vi "VelocityModeTestSDI.vi"() -> ()   [LabVIEW 2014]
uses:
  <resource>/objmgr/nimcca.rc
panel:
  in  "Velocity Setpoint":dbl
  in  "stop":bool
  out "error out":errorcluster
  in  "Motion Resource":refnum<k21>="nism://SoftMotionSDI9074/Axis 1"
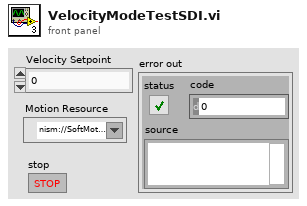
[diagram p1: front panel]
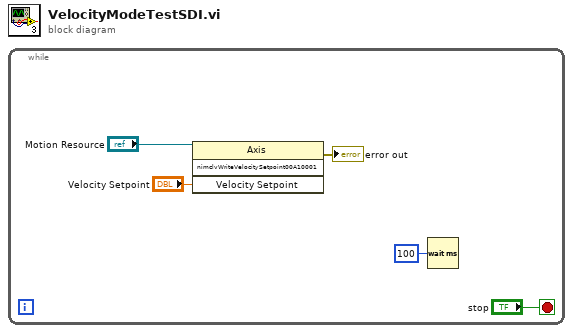
[diagram p0: block diagram]
diagram:
  n1 = while {
    stop <- "stop" stop-if-true
    n2 = invoke on="Invoke Node" class="Axis" method="nimclvWriteVelocitySetpoint00A10001"(reference="Motion Resource", "Velocity Setpoint"="Velocity Setpoint") -> (error out=→"error out":errorcluster)  [unwired: 2 in, 3 out]
    n3 = Wait (ms)(milliseconds to wait=u32 100) -> ()  [unwired: 1 out]
  }
